vi "Check Settings.vi"(8 "error in (no error)":errorcluster, 10 "Iterator Settings in":T1={"Prepare timeout (ms)"=200, "Iterate timeout (ms)"=50, "Conclude timeout (ms)"=200, "Iterate period (ms)"=200, "Number of iterations"=5, "Time before stop (ms)"=5, "Active Stop Conditions"={"Number of Iterations"=FALSE, "Time Elapsed"=FALSE, "Iteration Result"=FALSE}, "Prepare Msg"=refnum, "Iterate Msg"=refnum, "Conclude Msg"=refnum, "Iterations End Report"=refnum}, 11 "Abstract Iterator Actor in":refnum<class "Abstract Iterator Actor.lvclass">) -> (0 "error out":errorcluster, 2 "Iterator Settings out":T1={"Prepare timeout (ms)"=200, "Iterate timeout (ms)"=50, "Conclude timeout (ms)"=200, "Iterate period (ms)"=200, "Number of iterations"=5, "Time before stop (ms)"=5, "Active Stop Conditions"={"Number of Iterations"=FALSE, "Time Elapsed"=FALSE, "Iteration Result"=FALSE}, "Prepare Msg"=refnum, "Iterate Msg"=refnum, "Conclude Msg"=refnum, "Iterations End Report"=refnum}, 3 "Abstract Iterator Actor out":refnum<class "Abstract Iterator Actor.lvclass">)   [LabVIEW 2021, in "Iterator Actor.lvlib" / "Abstract Iterator Actor.lvclass"]
doc: "Checks the input settings of the iterator. \nReturns an error with a description if something is wrong."
uses:
  Abstract Iterator Actor.lvclass
  Iterator Settings.ctl
  Iterator Actor/Iterator Actor Abstract Messages/Iterator Report Iterations End Msg/Iterator Report Iterations End Msg.lvclass
  <vilib>/ActorFramework/Message/Message.lvclass
  Active Stop Conditions.ctl
  Iterator Errors.ctl
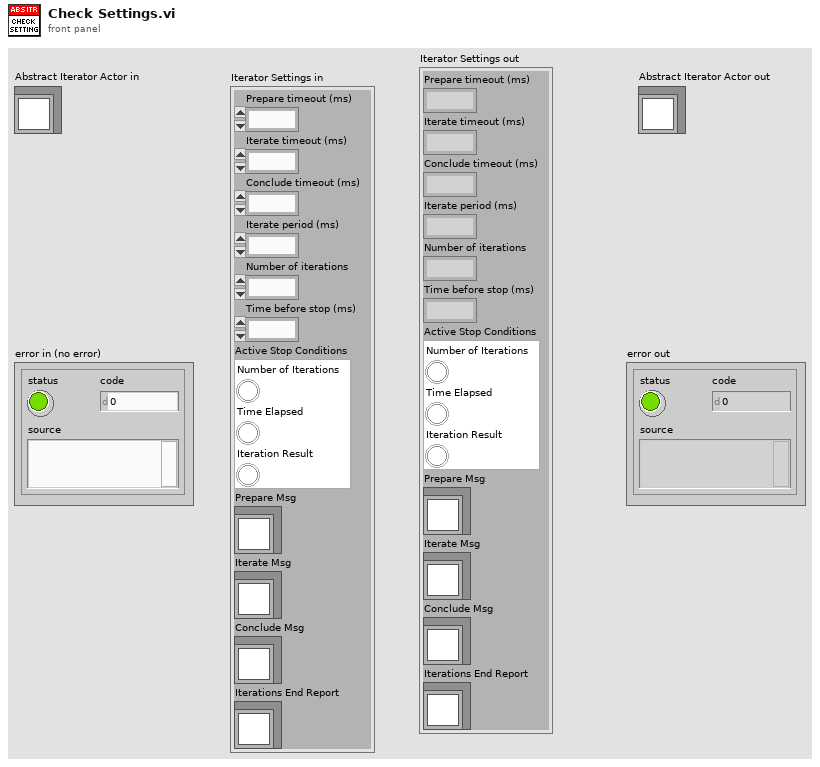
[diagram p1: front panel]
types:
  T1 = typedef "Iterator Actor.lvlib/Abstract Iterator Actor.lvclass/Iterator Settings.ctl" = cluster{"Prepare timeout (ms)":i32, "Iterate timeout (ms)":i32, "Conclude timeout (ms)":i32, "Iterate period (ms)":i32, "Number of iterations":i32, "Time before stop (ms)":i32, "Active Stop Conditions":T2, "Prepare Msg":refnum<class "Message.lvclass">, "Iterate Msg":refnum<class "Message.lvclass">, "Conclude Msg":refnum<class "Message.lvclass">, "Iterations End Report":refnum<class "Iterator Report Iterations End Msg.lvclass">}
  T2 = typedef "Iterator Actor.lvlib/Abstract Iterator Actor.lvclass/Active Stop Conditions.ctl" = cluster{"Number of Iterations":bool, "Time Elapsed":bool, "Iteration Result":bool}
  T3 = typedef "Iterator Actor.lvlib/Abstract Iterator Actor.lvclass/Stop Condition.ctl" = enum16{"None", "Number of Iterations", "Time Elapsed", "Iteration Result"}
  T4 = typedef "Iterator Actor.lvlib/Abstract Iterator Actor.lvclass/Iterator Errors.ctl" = enum16{"Input parameters are not valid", "Preparation call timed out", "Iteration call timed out", "Conclusion call timed out"}
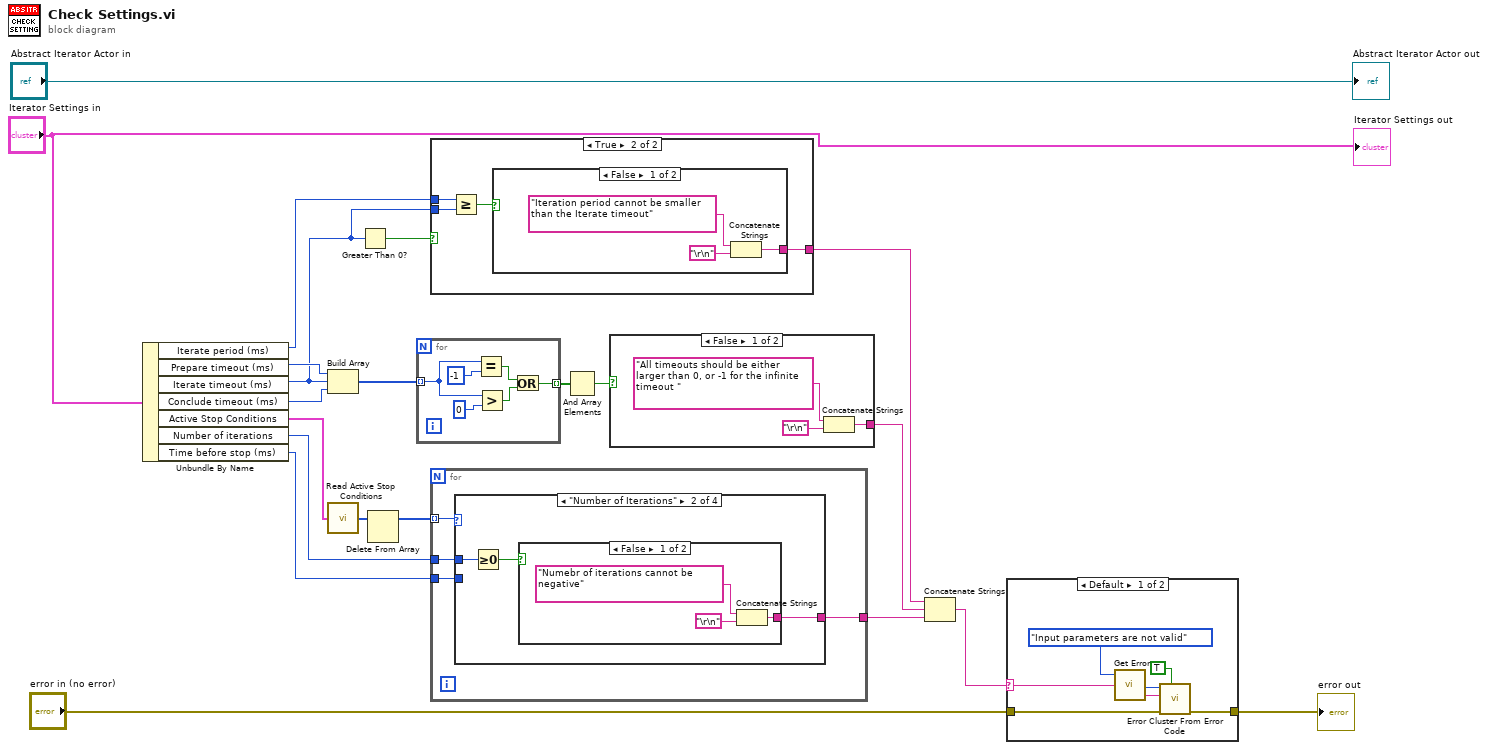
[diagram p0: block diagram]
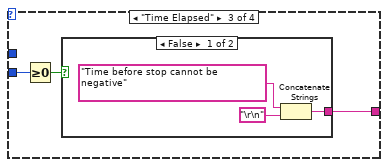
[diagram p4: hidden frame]
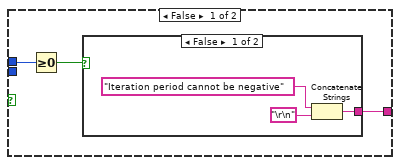
[diagram p7: hidden frame]
diagram:
  n1 = Unbundle By Name("Iterator Settings in") -> ("Iterate period (ms)"=w10:i32, "Prepare timeout (ms)"=w17:i32, "Iterate timeout (ms)"=w11:i32, "Conclude timeout (ms)"=w16:i32, "Active Stop Conditions"=w20:T2, "Number of iterations"=w9:i32, "Time before stop (ms)"=w8:i32)
  n2 = Build Array(w17, w11, w16) -> (w15:i32[])
  n3 = call "Read Active Stop Conditions.vi"("Active Stop Conditions"=w20) -> ("Active Stop Conditions"=w3:T3[])
  n4 = Greater Than 0?(x=w11) -> (x > 0?=w12:bool)
  n5 = Delete From Array(array=w3) -> (array with subset deleted=w2:T3[])  [unwired: 2 in, 1 out]
  n6 = for {
    tunnel: w15 -> [w25] mode=indexing
    tunnel: [w22] -> w14 mode=indexing
    n7 = Equal?(x=w25, y=-1) -> (x = y?=w23:bool)
    n8 = Greater?(x=w25, y=0) -> (0:w24:bool)
    n9 = Or(x=w23, y=w24) -> (x .or. y?=w22:bool)
  }
  n10 = case shown="True" w12 {
    tunnel: w11 -> [_ w37]
    tunnel: w10 -> [w30 w36]
    tunnel: [w28 w34] -> w5
    frame False {
      n11 = Greater Or Equal To 0?(x=w30) -> (x >= 0?=w29:bool)
      n12 = case shown="False" w29 {
        tunnel: [w32 _] -> w28
        frame False {
          n13 = Concatenate Strings("Iteration period cannot be negative", "\r\n") -> (w32:string)
        }
        frame True {
        }
      }
    }
    frame True {
      n14 = Greater Or Equal?(x=w36, y=w37) -> (x >= y?=w35:bool)
      n15 = case shown="False" w35 {
        tunnel: [w38 _] -> w34
        frame False {
          n16 = Concatenate Strings("Iteration period cannot be smaller than the Iterate timeout", "\r\n") -> (w38:string)
        }
        frame True {
        }
      }
    }
  }
  n17 = for {
    tunnel: w2 -> [w44] mode=indexing
    tunnel: w9 -> [w43]
    tunnel: w8 -> [w42]
    tunnel: [w41] -> w7
    n18 = case shown="\"Number of Iterations\"" w44 {
      tunnel: w43 -> [_ w47 _ _]
      tunnel: w42 -> [_ _ w53 _]
      tunnel: [_ w45 w51 _] -> w41
      frame "None", Default {
      }
      frame "Number of Iterations" {
        n19 = Greater Or Equal To 0?(x=w47) -> (x >= 0?=w46:bool)
        n20 = case shown="False" w46 {
          tunnel: [w49 _] -> w45
          frame False {
            n21 = Concatenate Strings("Numebr of iterations cannot be negative", "\r\n") -> (w49:string)
          }
          frame True {
          }
        }
      }
      frame "Time Elapsed" {
        n22 = Greater Or Equal To 0?(x=w53) -> (x >= 0?=w52:bool)
        n23 = case shown="False" w52 {
          tunnel: [w54 _] -> w51
          frame False {
            n24 = Concatenate Strings("Time before stop cannot be negative", "\r\n") -> (w54:string)
          }
          frame True {
          }
        }
      }
      frame "Iteration Result" {
      }
    }
  }
  n25 = And Array Elements(Boolean array=w14) -> (logical AND=w13:bool)
  n26 = case shown="False" w13 {
    tunnel: [w57 _] -> w6
    frame False {
      n27 = Concatenate Strings("All timeouts should be either larger than 0, or -1 for the infinite timeout ", "\r\n") -> (w57:string)
    }
    frame True {
    }
  }
  n28 = Concatenate Strings(w5, w6, w7) -> (w4:string)
  n29 = case shown="Default" w4 {
    selector: w4 -> [w60 _]
    tunnel: "error in (no error)" -> [w63 w67]
    tunnel: [w62 w67] -> w19
    frame Default {
      n30 = call "Get Error.vi"("Error Additional Information"=w60, "Error"=Iterator_Errors."Input parameters are not valid") -> ("source"=w65:string, "code"=w64:i32)  [unwired: 1 in, 1 out]
      n31 = call <vilib>:"Error Cluster From Error Code.vi"("show call chain? (False)"=TRUE ("is warning? (False)"), "error in (no error)"=w63, "error message (\"\")"=w65, "error code (0)"=w64) -> ("error out"=w62:errorcluster)  [unwired: 5 in]
    }
    frame "" {
    }
  }
  "error out" <- w19
  "Abstract Iterator Actor out" <- "Abstract Iterator Actor in"
  "Iterator Settings out" <- "Iterator Settings in"
